vi "toml_example.vi"() -> ()   [LabVIEW 2017]
uses:
  toml/toml.llb/toml_value_operation.ctl
panel:
  out "error out":errorcluster
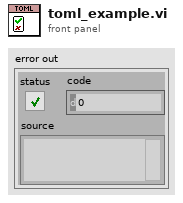
[diagram p1: front panel]
types:
  T1 = typedef "toml_value_operation.ctl" = enum8{"read", "write"}
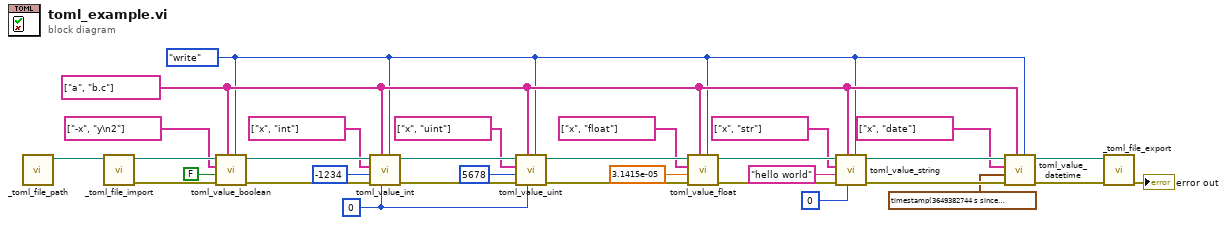
[diagram p0: block diagram]
diagram:
  w18 = u16 0 ("modifiers")
  w4 = string[] ["a", "b.c"] ("section")
  w3 = toml_value_operation."write" ("operation")
  n1 = call "_toml_file_path.vi"() -> ("app toml path"=w32:path)  [unwired: 8 in, 3 out]
  n2 = call "_toml_file_import.vi"("path in"=w32) -> ("error out"=w31:errorcluster, "path out"=w30:path)  [unwired: 9 in]
  n3 = call "toml_value_boolean.vi"("operation"=w3, "section"=w4, "error in (no error)"=w31, "value in"=FALSE, "key"=string[] ["-x", "y\n2"], "path in"=w30) -> ("error out"=w25:errorcluster, "path out"=w23:path)  [unwired: 2 in, 2 out]
  n4 = call "toml_value_int.vi"("operation"=w3, "modifiers"=w18, "section"=w4, "error in (no error)"=w25, "value in"=i64 -1234, "key"=string[] ["x", "int"], "path in"=w23) -> ("error out"=w26:errorcluster, "path out"=w24:path)  [unwired: 1 in, 2 out]
  n5 = call "toml_value_uint.vi"("operation"=w3, "modifiers"=w18, "section"=w4, "error in (no error)"=w26, "value in"=u64 5678, "key"=string[] ["x", "uint"], "path in"=w24) -> ("error out"=w17:errorcluster, "path out"=w16:path)  [unwired: 1 in, 2 out]
  n6 = call "toml_value_float.vi"("operation"=w3, "section"=w4, "error in (no error)"=w17, "value in"=3.1415e-05, "key"=string[] ["x", "float"], "path in"=w16) -> ("error out"=w13:errorcluster, "path out"=w12:path)  [unwired: 2 in, 2 out]
  n7 = call "toml_value_string.vi"("operation"=w3, "modifiers"=u16 0, "section"=w4, "error in (no error)"=w13, "value in"="hello world", "key"=string[] ["x", "str"], "path in"=w12) -> ("error out"=w8:errorcluster, "path out"=w6:path)  [unwired: 1 in, 2 out]
  n8 = call "toml_value_datetime.vi"("operation"=w3, "section"=w4, "error in (no error)"=w8, "value in"=timestamp(3649382744.631476 s since 1904-01-01), "key"=string[] ["x", "date"], "path in"=w6) -> ("error out"=w7:errorcluster, "path out"=w5:path)  [unwired: 2 in, 2 out]
  n9 = call "_toml_file_export.vi"("error in (no error)"=w7, "path in"=w5) -> ("error out"=→"error out":errorcluster)  [unwired: 8 in, 1 out]
